vi "REVION_VI.vi"(8 "ERRIN":errorcluster caption="entrée d'erreur (pas d'erreur)") -> (0 "ERROUT":errorcluster caption="sortie d'erreur", 3 "N° Révision":u32)   [LabVIEW 2020]
uses:
  VG/Revision.vi
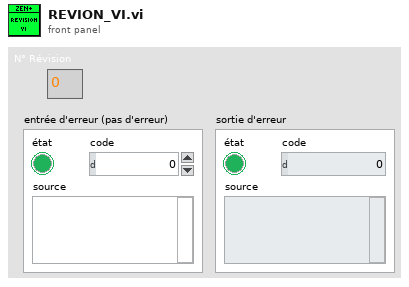
[diagram p1: front panel]
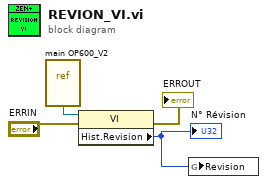
[diagram p0: block diagram]
diagram:
  n1 = vi-ref "main OP600_V2.vi"() -> (w2:refnum<vi>)
  n2 = property class="VI"(reference=w2, error in="ERRIN") -> (error out=→"ERROUT":errorcluster, "Hist.Revision"=w4:u32)  [unwired: 1 out]
  "N° Révision" <- w4
  n3 = global write "Revision.vi" "Revision"(w4) -> ()
